vi "To JSON.vi"(8 "error in":errorcluster, 11 "PDO Communication Parameter in":refnum<class "PDO Communication Parameter.lvclass">) -> (0 "error out":errorcluster, 2 "<JSON>":string, 3 "PDO Communication Parameter out":refnum<class "PDO Communication Parameter.lvclass">)   [LabVIEW 2020, in "CANopen.lvlib" / "PDO Communication Parameter.lvclass"]
uses:
  PDO Communication Parameter.lvclass
  PDO Communication Parameter.lvclass/PDO Communication Parameter.ctl
  5766efa4-6552-4b53-84aa-e97d7a73cf22.vi
  ad16f34d-1780-4a34-aa17-0f388abc6a8c.vi
  806c50ae-49b5-48fd-a660-cb2f8af3051b.vi
  <vilib>/JDP Science/JSONtext/Variant to JSON Text.vi
  <vilib>/JDP Science/JSONtext/Set Multiple Object Items.vi
  <vilib>/JDP Science/JSONtext/LVClass Serializer/JSONtext LVClass Serializer.lvclass
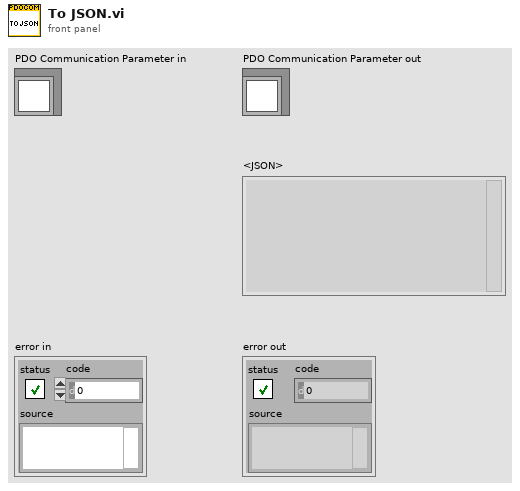
[diagram p1: front panel]
types:
  T1 = typedef "CANopen.lvlib/Access Type.ctl" = enum16{"unknown", "ro", "wo", "rw", "rwr", "rww", "const"}
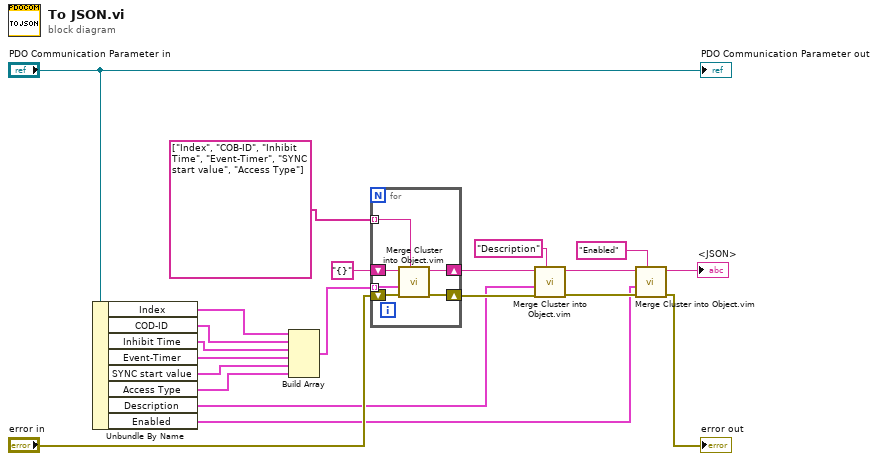
[diagram p0: block diagram]
diagram:
  n1 = Unbundle By Name("PDO Communication Parameter in") -> ("Index"=w18:cluster{"Null":bool, "Value":u16}, "COD-ID"=w17:cluster{"Null":bool, "Value":u32}, "Inhibit Time"=w16:cluster{"Null":bool, "Value":u16}, "Event-Timer"=w15:cluster{"Null":bool, "Value":u16}, "SYNC start value"=w14:cluster{"Null":bool, "Value":u8}, "Access Type"=w13:cluster{"Null":bool, "Value":T1}, "Description"=w8:cluster{"Null":bool, "Value":string}, "Enabled"=w6:cluster{"Null":bool, "Value":bool})
  n2 = Build Array(w18, w17, w16, w15, w14, w13) -> (w12:cluster{"Null":bool, "Value":u32}[])
  n3 = for {
    shift-right: [w25] -> w10
    shift-left: "{}" -> [w26]
    tunnel: string[] ["Index", "COB-ID", "Inhibit Time", "Event-Timer", "SYNC start value", "Access Type"] -> [w27] mode=indexing
    tunnel: w12 -> [w24] mode=indexing
    shift-right: [w22] -> w9
    shift-left: "error in" -> [w23]
    n4 = call "Merge Cluster into Object.vim"("$Path or Item Name"=w27, "error in (no error)"=w23, "Any Cluster"=w24, "JSON"=w26) -> ("error out"=w22:errorcluster, "<JSON>"=w25:string)  [unwired: 5 in]
  }
  n5 = call "Merge Cluster into Object.vim"("$Path or Item Name"="Description", "error in (no error)"=w9, "Any Cluster"=w8, "JSON"=w10) -> ("error out"=w7:errorcluster, "<JSON>"=w5:string)  [unwired: 5 in]
  n6 = call "Merge Cluster into Object.vim"("$Path or Item Name"="Enabled", "error in (no error)"=w7, "Any Cluster"=w6, "JSON"=w5) -> ("error out"=→"error out":errorcluster, "<JSON>"=→"<JSON>":string)  [unwired: 5 in]
  "PDO Communication Parameter out" <- "PDO Communication Parameter in"
